vi "from string 3.2.vi"(8 "error in":errorcluster, 10 "data in":string, 11 "Shared Memory configuration in":refnum<class "Shared Memory configuration.lvclass">) -> (0 "error out":errorcluster, 2 "remaining data":string, 3 "Shared Memory configuration out":refnum<class "Shared Memory configuration.lvclass">)   [LabVIEW 2014, in "Shared Memory configuration.lvclass"]
uses:
  Shared Memory configuration.lvclass
  Shared Memory configuration.lvclass/Shared Memory configuration.ctl
  <vilib>/NI/Configuration Framework/serializable configuration/NISE_CEF_serializable configuration.lvclass
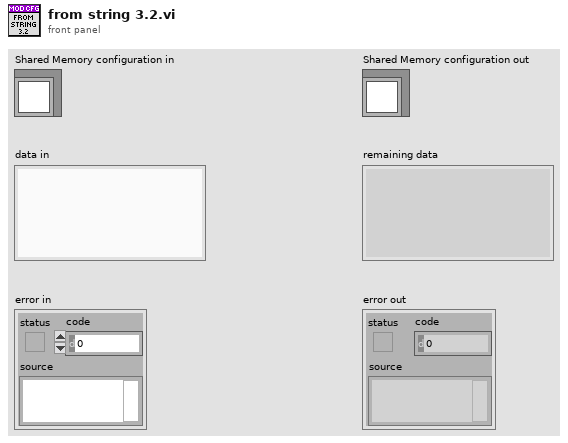
[diagram p1: front panel]
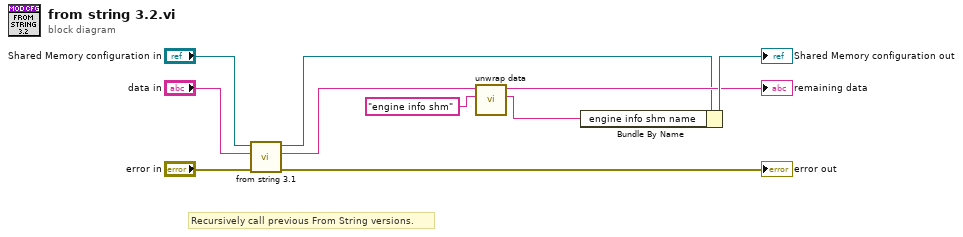
[diagram p0: block diagram]
diagram:
  # "Recursively call previous From String versions."
  n1 = call "from string 3.1.vi"("error in"="error in", "data in"="data in", "Shared Memory configuration in"="Shared Memory configuration in") -> ("error out"=→"error out":errorcluster, "remaining data"=w2:string, "Shared Memory configuration out"=w4:refnum<class "Shared Memory configuration.lvclass">)  [unwired: 6 in]
  n2 = call <vilib>:"unwrap data.vi"("identifier"="engine info shm", "data to unwrap"=w2) -> ("unwrapped data"=w1:string, "remaining string"=→"remaining data":string)  [unwired: 8 in]
  n3 = Bundle By Name(cluster=w4, "engine info shm name"=w1) -> (→"Shared Memory configuration out":refnum<class "Shared Memory configuration.lvclass">)
